vi "small current measurement.vi"() -> ()   [LabVIEW 2016, in "features.lvlib"]
doc: "This vi shows all current measurements in small format"
uses:
  Features/features/features.lvlib
  sub-VIs/sub-VIs.lvlib
panel:
  in  "Tab Control":enum32{"Measurements", "Errors"}(tab)
  out "cup being read":string
  out "Current measurements":dbl(graph)
  out "Current":dbl format="%#_4p"
  in  "stop":bool
  out "switch cup position?":bool
  out "offset cup Actual":dbl format="%#_5g"
  out "VI error":errorcluster
  out "inj current":dbl format="%#_3p"
  out "rare count rate read error":errorcluster
  out "Inj current SV read error":errorcluster
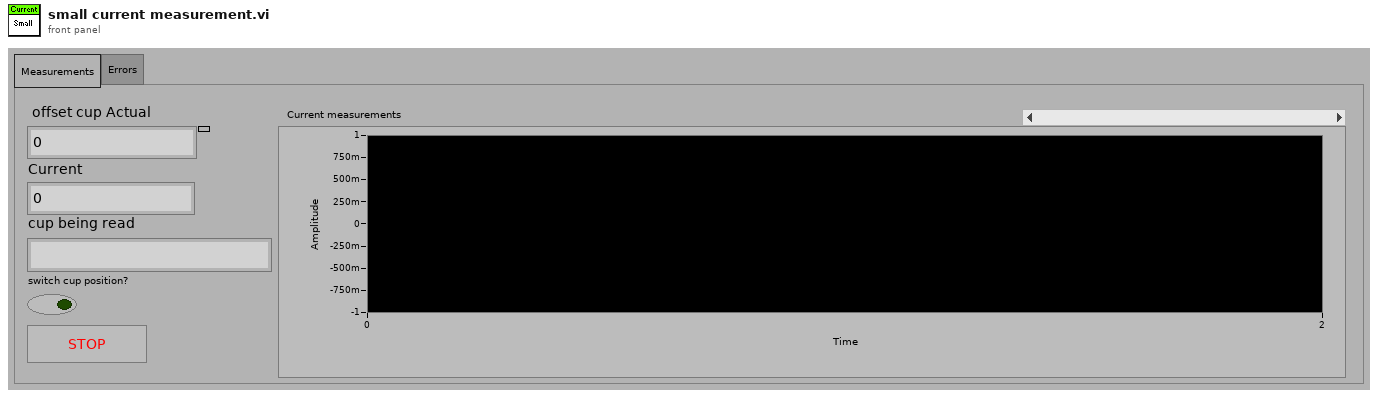
[diagram p1: front panel]
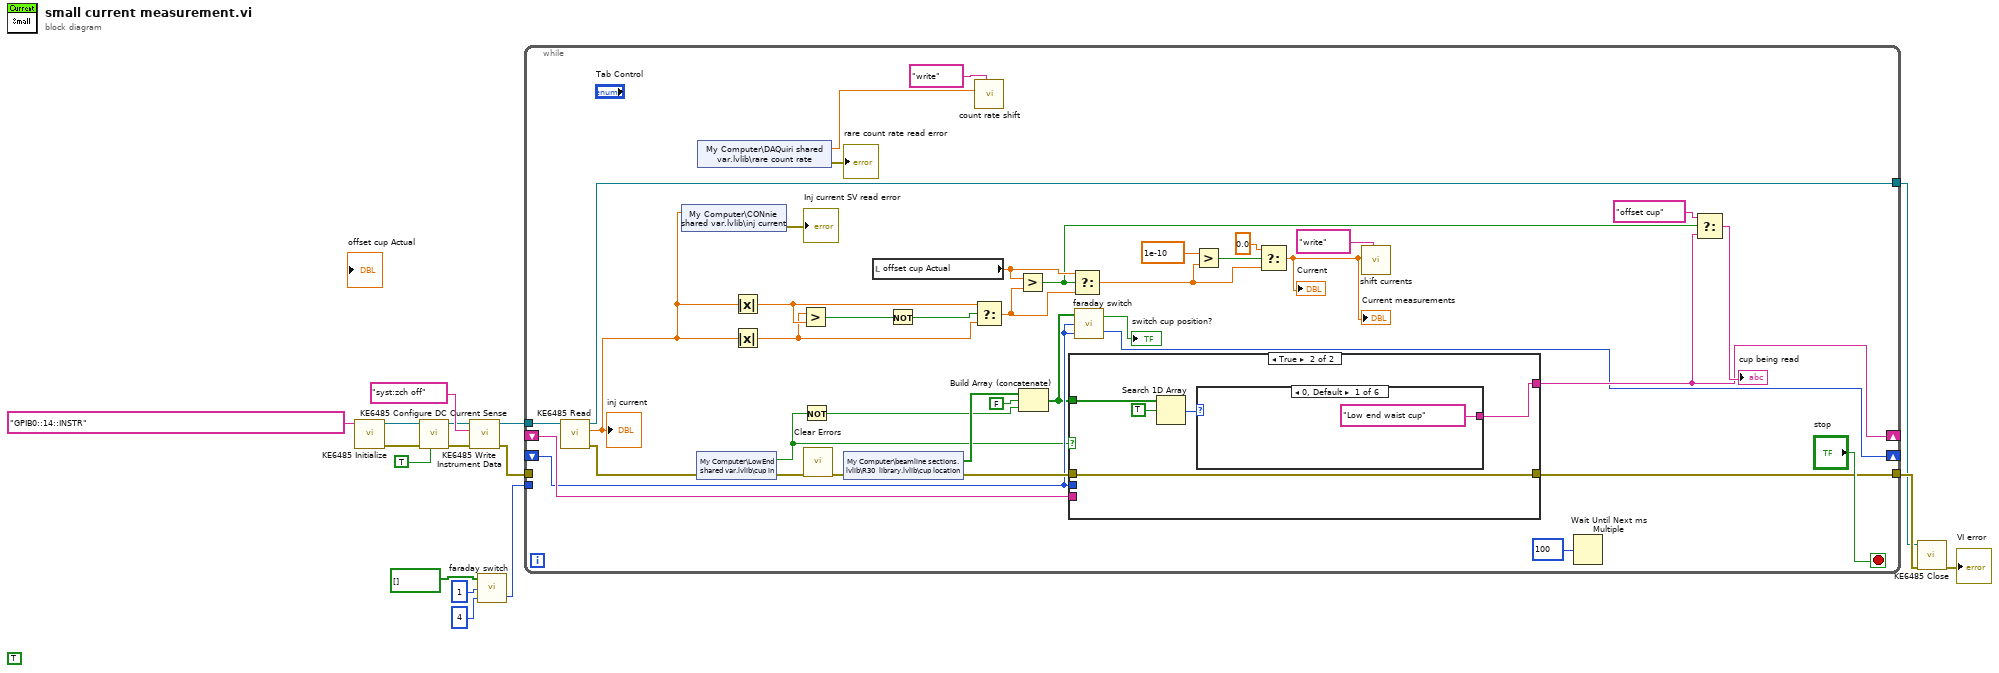
[diagram p0: block diagram]
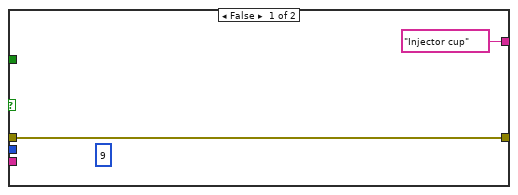
[diagram p2: hidden frame]
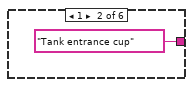
[diagram p3: hidden frame]
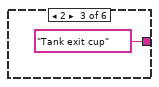
[diagram p4: hidden frame]
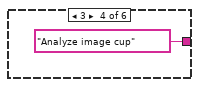
[diagram p5: hidden frame]
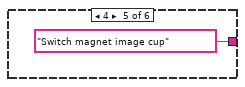
[diagram p6: hidden frame]
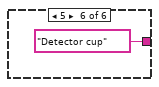
[diagram p7: hidden frame]
diagram:
  (unwired) TRUE ("autorange")
  n1 = call "KE6485 Initialize.vi"("resource name"="GPIB0::14::INSTR") -> ("error out"=w13:errorcluster, "instrument handle out"=w12:refnum<k15>)  [unwired: 3 in, 6 out]
  n2 = call "KE6485 Configure DC Current Sense.vi"("autorange"=TRUE, "error in (no error)"=w13, "instrument handle"=w12) -> ("error out"=w15:errorcluster, "instrument handle out"=w14:refnum<k15>)  [unwired: 3 in, 4 out]
  n3 = call "KE6485 Write Instrument Data.vi"("error in (no error)"=w15, "write buffer"="syst:zch off" ("resource name"), "instrument handle"=w14) -> ("error out"=w9:errorcluster, "instrument handle out"=w10:refnum<k15>)  [unwired: 7 out]
  n4 = call "faraday switch.vi"("cup position"=4, "index in"=1, "input fc array"=bool[] []) -> ("index out"=w2:i32)  [unwired: 1 out]
  n5 = while {
    tunnel: w10 -> [w53]
    tunnel: w9 -> [_]
    tunnel: [w41] -> w7
    tunnel: [w21] -> w6
    shift-right: [w30] -> _
    shift-left: _ -> [w29]
    shift-right: [w28] -> _
    shift-left: _ -> [w23]
    tunnel: w2 -> [_]
    stop <- "stop" stop-if-true
    n6 = call "KE6485 Read.vi"("instrument handle"=w53) -> ("error out"=w45:errorcluster, "reading"=w24:dbl, "instrument handle out"=w21:refnum<k15>)  [unwired: 2 in, 6 out]
    "inj current" <- w24
    n7 = shared-variable "My Computer\\CONnie shared var.lvlib\\inj current"(w24) -> (error out=→"Inj current SV read error":errorcluster)  [unwired: 1 in]
    n8 = shared-variable "My Computer\\LowEnd shared var.lvlib\\cup in"(error in=w45) -> (w18:bool, error out=w44:errorcluster)
    n9 = shared-variable "My Computer\\DAQuiri shared var.lvlib\\rare count rate"() -> (w33:dbl, error out=→"rare count rate read error":errorcluster)  [unwired: 1 in]
    n10 = Absolute Value(x=w24) -> (abs(x)=w47:dbl)
    n11 = Absolute Value(x=w24) -> (abs(x)=w46:dbl)
    n12 = Greater?(x=w46, y=w47) -> (0:w49:bool)
    n13 = Not(x=w18) -> (.not. x?=w17:bool)
    n14 = call <vilib>:"Clear Errors.vi"("error in (no error)"=w44) -> ("error out"=w26:errorcluster)  [unwired: 1 in, 5 out]
    n15 = shared-variable "My Computer\\beamline sections.lvlib\\R30  library.lvlib\\cup location"(error in=w26) -> (w22:bool[], error out=w25:errorcluster)
    n16 = local read "offset cup Actual"() -> (w39:dbl)
    n17 = Not(x=w49) -> (.not. x?=w48:bool)
    n18 = call "count rate shift.vi"("read or write"="write" ("Combo Box"), "count rate in"=w33) -> ()  [unwired: 9 in, 1 out]
    n19 = Select(t=w47, s=w48, f=w46) -> (s? t:f=w40:dbl)
    n20 = Greater?(x=w39, y=w40) -> (0:w37:bool)
    n21 = Build Array (concatenate)(w22, FALSE ("Boolean"), w17) -> (w19:bool[])
    n22 = case shown="True" w18 {
      tunnel: ["Injector cup" ("cup being read") w60] -> w30
      tunnel: w25 -> [w57 w58]
      tunnel: [w57 w58] -> w41
      tunnel: w29 -> [_ _]
      tunnel: w19 -> [_ w59]
      tunnel: w23 -> [_ _]
      frame False {
        (unwired) 9 ("index out")
      }
      frame True {
        n23 = Search 1D Array(1D array=w59, element=TRUE) -> (index of element=w61:i32)  [unwired: 1 in]
        n24 = case shown="0, Default" w61 {
          tunnel: ["Low end waist cup" ("cup being read") "Tank entrance cup" ("cup being read") "Tank exit cup" ("cup being read") "Analyze image cup" ("cup being read") "Switch magnet image cup" ("cup being read") "Detector cup" ("cup being read")] -> w60
          frame 0, Default {
          }
          frame 1 {
          }
          frame 2 {
          }
          frame 3 {
          }
          frame 4 {
          }
          frame 5 {
          }
        }
      }
    }
    n25 = Select(t=w39, s=w37, f=w40) -> (s? t:f=w38:dbl)
    n26 = call "faraday switch.vi"("cup position"=w23, "index in"=w23, "input fc array"=w19) -> ("index out"=w28:i32, "switch cup position?"=→"switch cup position?":bool)
    n27 = Greater?(x=1e-10, y=w38) -> (0:w51:bool)
    n28 = Select(t=0.0, s=w51, f=w38) -> (s? t:f=w42:dbl)
    "Current" <- w42
    "Current measurements" <- w42
    n29 = call "shift currents.vi"("Combo Box"="write", "current in"=w42) -> ()  [unwired: 9 in, 1 out]
    n30 = Wait Until Next ms Multiple(millisecond multiple=u32 100) -> ()  [unwired: 1 out]
    n31 = Select(t="offset cup", s=w37, f=w30) -> (s? t:f=→"cup being read":string)
  }
  n32 = call "KE6485 Close.vi"("error in (no error)"=w7, "instrument handle"=w6) -> ("error out"=→"VI error":errorcluster)  [unwired: 9 out]
